vi "irradiance 1030 - run only.vi"(11 "Boolean":bool) -> (10 "Irradiance":dbl)   [LabVIEW 2021]
uses:
  irradiance 1030_global variable.vi
panel:
  in  "Pyranometer sensitivity (µV/W/m²) 2":dbl=7.02e-05
  out "Pyranometer - Waveform Chart 2":dbl(graph)
  in  "Measurements per channel 2":i32=3 min=1 max=1000
  in  "Measurement channels 2":string="1030"
  in  "VISA resource name":refnum<visa-resource-name>="USB0::2391::1287::MY44008368::0::INSTR"
  in  "error in (no error)":errorcluster
  out "VISA/Instrument Errors":errorcluster
  # "TO DO\n- automatically update date at every reading\n- append new reading to the same file\n- take mean of multiple readings"
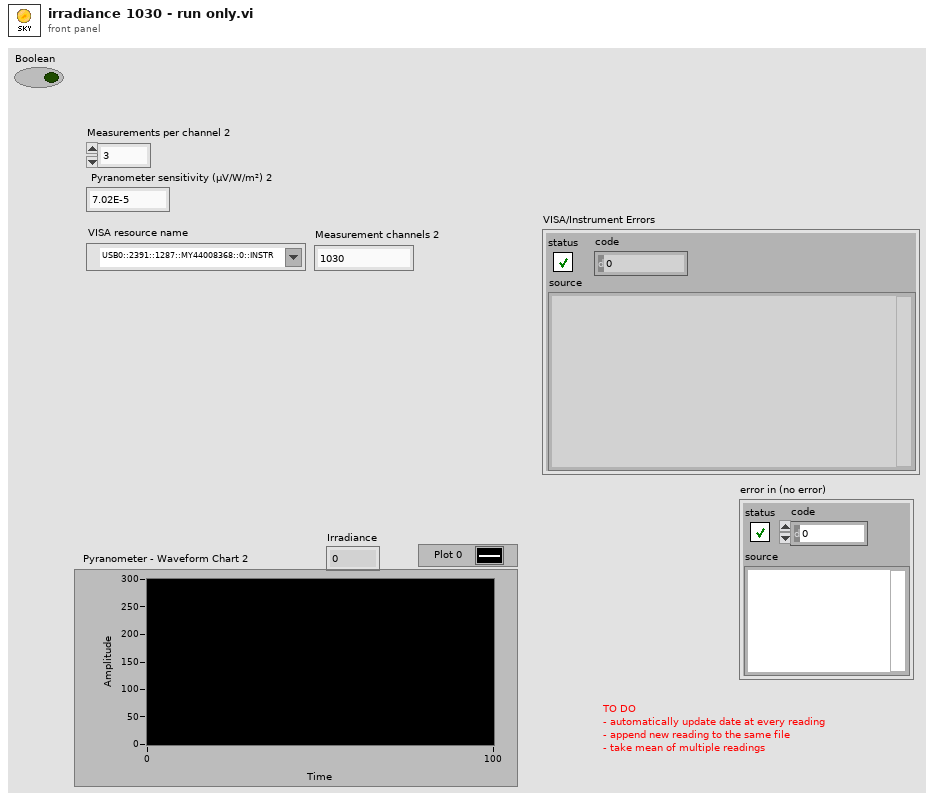
[diagram p1: front panel]
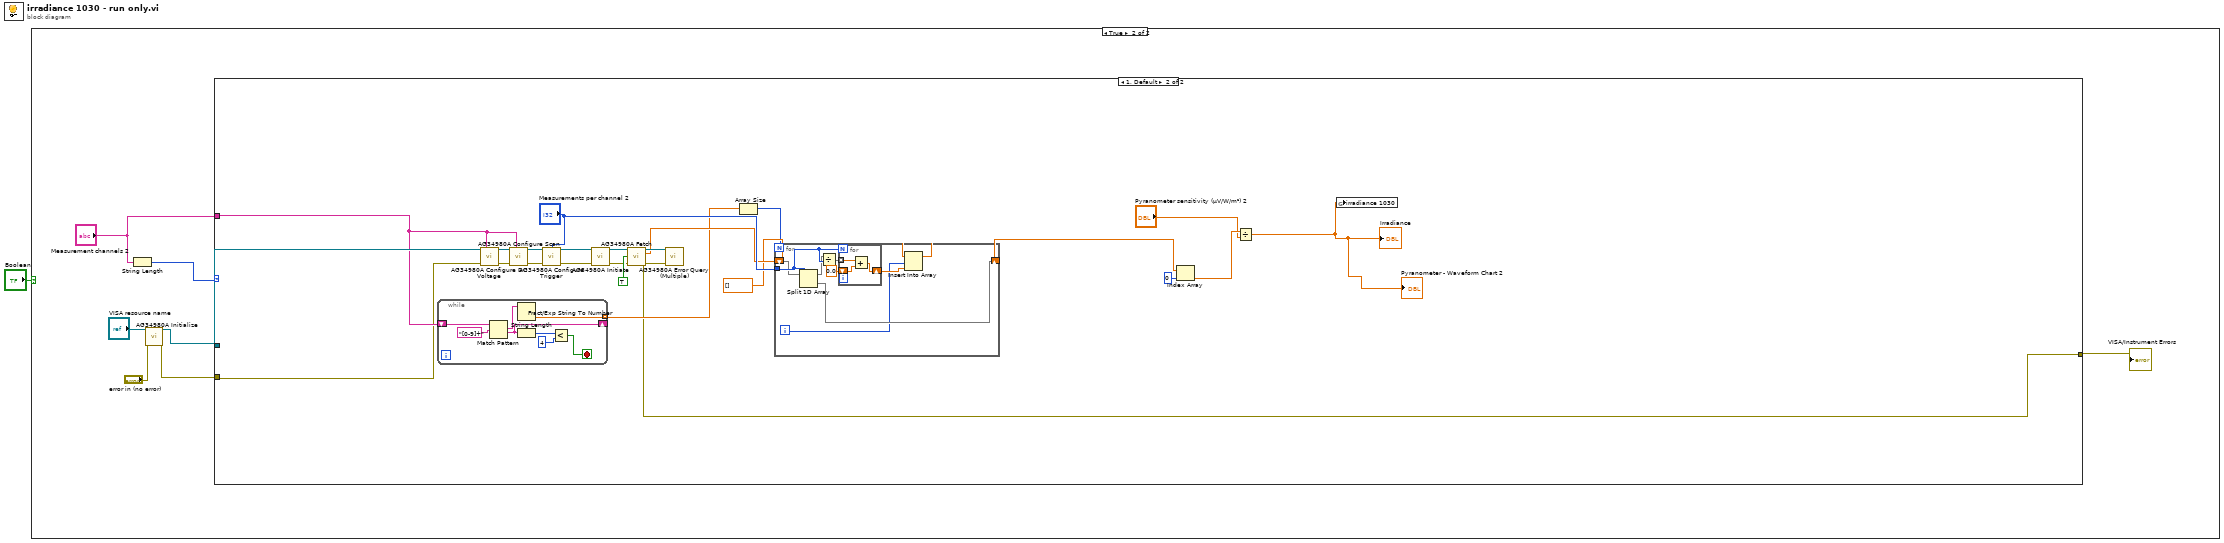
[diagram p0: block diagram]
diagram:
  n1 = case shown="True" "Boolean" {
    frame False {
    }
    frame True {
      n2 = String Length(string="Measurement channels 2") -> (length=w4:i32)
      n3 = call "AG34980A Initialize.vi"("VISA resource name"="VISA resource name", "error in (no error)"="error in (no error)") -> ("VISA session"=w3:refnum<visa-resource-name>, "error out"=w2:errorcluster)  [unwired: 12 in]
      n4 = case shown="1, Default" w4 {
        tunnel: [w9 w10] -> w8
        tunnel: w3 -> [_ w34]
        tunnel: "Measurement channels 2" -> [_ w33]
        tunnel: w2 -> [w9 w12]
        frame 0 {
        }
        frame 1, Default {
          n5 = while {
            shift-right: [w48] -> _
            shift-left: w33 -> [w51]
            tunnel: [w50] -> w17 mode=indexing
            stop <- w49 stop-if-true
            n6 = Match Pattern(string=w51, regular expression="[0-9]+" ("Thermocouple channels")) -> (match substring=w55:string, after substring=w48:string)  [unwired: 1 in, 2 out]
            n7 = Fract/Exp String To Number(string=w55) -> (number=w50:dbl)  [unwired: 3 in, 1 out]
            n8 = String Length(string=w48) -> (length=w53:i32)
            n9 = Less?(x=w53, y=4) -> (x < y?=w49:bool)
          }
          n10 = call "AG34980A Configure DC Voltage.vi"("VISA resource name"=w34, "Channel List(empty)"=w33, "error in (no error)"=w12) -> ("VISA resource name out"=w32:refnum<visa-resource-name>, "error out"=w26:errorcluster)  [unwired: 11 in]
          n11 = call "AG34980A Configure Scan.vi"("VISA resource name"=w32, "Scan List(empty)"=w33, "error in (no error)"=w26) -> ("VISA resource name out"=w31:refnum<visa-resource-name>, "error out"=w25:errorcluster)  [unwired: 11 in]
          n12 = call "AG34980A Configure Trigger.vi"("VISA resource name"=w31, "Sample Count (1)"="Measurements per channel 2", "error in (no error)"=w25) -> ("VISA resource name out"=w30:refnum<visa-resource-name>, "error out"=w24:errorcluster)  [unwired: 11 in]
          n13 = call "AG34980A Initiate.vi"("VISA resource name"=w30, "error in (no error)"=w24) -> ("VISA resource name out"=w29:refnum<visa-resource-name>, "error out"=w23:errorcluster)  [unwired: 12 in]
          n14 = call "AG34980A Fetch.vi"("VISA resource name"=w29, "Numbers Only (T:On)"=TRUE, "error in (no error)"=w23) -> ("VISA resource name out"=w28:refnum<visa-resource-name>, "Output Data (Numbers Only)"=w20:dbl[], "error out"=w22:errorcluster)  [unwired: 9 in, 1 out]
          n15 = call "AG34980A Error Query (Multiple).vi"("VISA resource name"=w28, "error in (no error)"=w22) -> ("error out"=w10:errorcluster)  [unwired: 10 in, 3 out]
          n16 = Array Size(array=w17) -> (size(s)=w18:i32)
          n17 = for {
            N: w18 -> [_]
            shift-right: [w44] -> _
            shift-left: w20 -> [w36]
            shift-right: [w38] -> w14
            shift-left: dbl[] [] -> [w39]
            tunnel: "Measurements per channel 2" -> [w37]
            i -> [w40]
            n18 = Split 1D Array(array=w36, index=w37) -> (first subarray=w35:dbl[], second subarray=w44:dbl[])
            n19 = Divide(x=w35, y=w37) -> (x/y=w42:dbl[])
            n20 = for {
              N: w37 -> [_]
              shift-right: [w45] -> w41
              shift-left: 0.0 ("index") -> [w47]
              tunnel: w42 -> [w46] mode=indexing
              n21 = Add(x=w46, y=w47) -> (x+y=w45:dbl)
            }
            n22 = Insert Into Array(array=w39, index=w40, new element=w41) -> (w38:dbl[])
          }
          n23 = Index Array(array=w14, index=0) -> (element=w15:dbl)
          n24 = Divide(x=w15, y="Pyranometer sensitivity (µV/W/m²) 2") -> (x/y=w11:dbl)
          "Pyranometer - Waveform Chart 2" <- w11
          "Irradiance" <- w11
          n25 = global write "irradiance 1030_global variable.vi" "irradiance 1030"(w11) -> ()
        }
      }
      "VISA/Instrument Errors" <- w8
    }
  }
